vi "Explain Error (Improved) UI.vi"(8 "User VI Ref":refnum<vi>, 9 "Error Cluster":errorcluster) -> ()   [LabVIEW 2020, in "Explain Error Improved Dialog.lvlib"]
uses:
  Explain Error Improved Dialog/Explain Error Improved Dialog.lvlib
  <vilib>/Utility/error.llb/DialogTypeEnum.ctl
  <vilib>/Utility/error.llb/DialogType.ctl
  <vilib>/Platform/browser.llb/Open URL in Default Browser (string).vi
  <vilib>/Utility/inputDevices.llb/mouseAcquire.vi
  <vilib>/Utility/inputDevices.llb/keyboardAcquire.vi
  <vilib>/Utility/cursorutil.llb/Set Cursor (Icon Pict).vi
  <vilib>/Utility/inputDevices.llb/closeKeyboard.vi
  <vilib>/Utility/inputDevices.llb/closeMouse.vi
  fc0d4d85-7f14-4b45-b7f8-c4820347555e.vi
panel:
  in  "search google":bool
  out "Explanation":string
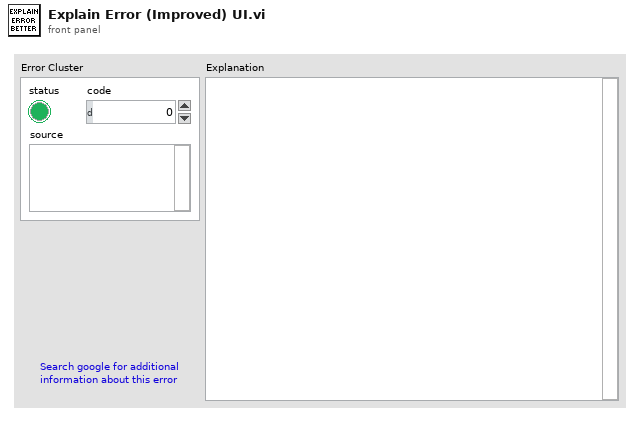
[diagram p1: front panel]
types:
  T1 = typedef "DialogTypeEnum.ctl" = enum16{"no dialog", "OK message", "continue or stop message", "auto error handling dialog", "OK message + warnings", "continue/stop + warnings"}
  T2 = typedef "DialogType.ctl" = u16
  T3 = cluster{"vi name":string, "start":i32, "end":i32}[]
  T4 = typedef "LVPoint32TypeDef.ctl" = cluster{"Horizontal":i32, "Vertical":i32}
  T5 = cluster{"button 1":bool, "button 2":bool, "button 3":bool, "button 4":bool}
  T6 = cluster{"vi name":string, "start":i32, "end":i32}
  T7 = enum16{"0", "1", "2", "3", "4", "5", "6", "7", "8", "9", "A", "B", "C", "D", "E", "F", "G", "H", "I", "J", "K", "L", "M", "N", "O", "P", "Q", "R", "S", "T", "U", "V", "W", "X", "Y", "Z", "F1", "F2", "F3", "F4", "F5", "F6", "F7", "F8", "F9", "F10", "F11", "F12", "F13", "F14", "F15", "ADD", "BACK", "BACKSLASH", "CAPITAL", "COMMA", "DECIMAL", "DELETE", "DIVIDE", "DOWN", "END", "EQUALS", "ESCAPE", "GRAVE (`)", "HOME", "INSERT", "LBRACKET", "LCONTROL", "LEFT", "L ALT", "LSHIFT", "LWIN", "MINUS", "MULTIPLY", "NEXT", "NUMLOCK", "NUMPAD_0", "NUMPAD_1", "NUMPAD_2", "NUMPAD_3", "NUMPAD_4", "NUMPAD_5", "NUMPAD_6", "NUMPAD_7", "NUMPAD_8", "NUMPAD_9", "PAUSE", "PERIOD", "PRIOR (PG UP)", "RBRACKET", "RCONTROL", "RETURN", "RIGHT", "R ALT", "RSHIFT", "RWIN", "SCROLL", "SEMICOLON", "SLASH", "SPACE", "SUBTRACT", "TAB", "UP", "ENTER (num pad)", "' (quote)"}[]
  T8 = cluster{"Shift":bool, "Ctrl":bool, "Alt":bool, "Cmd":bool, "Opt":bool}
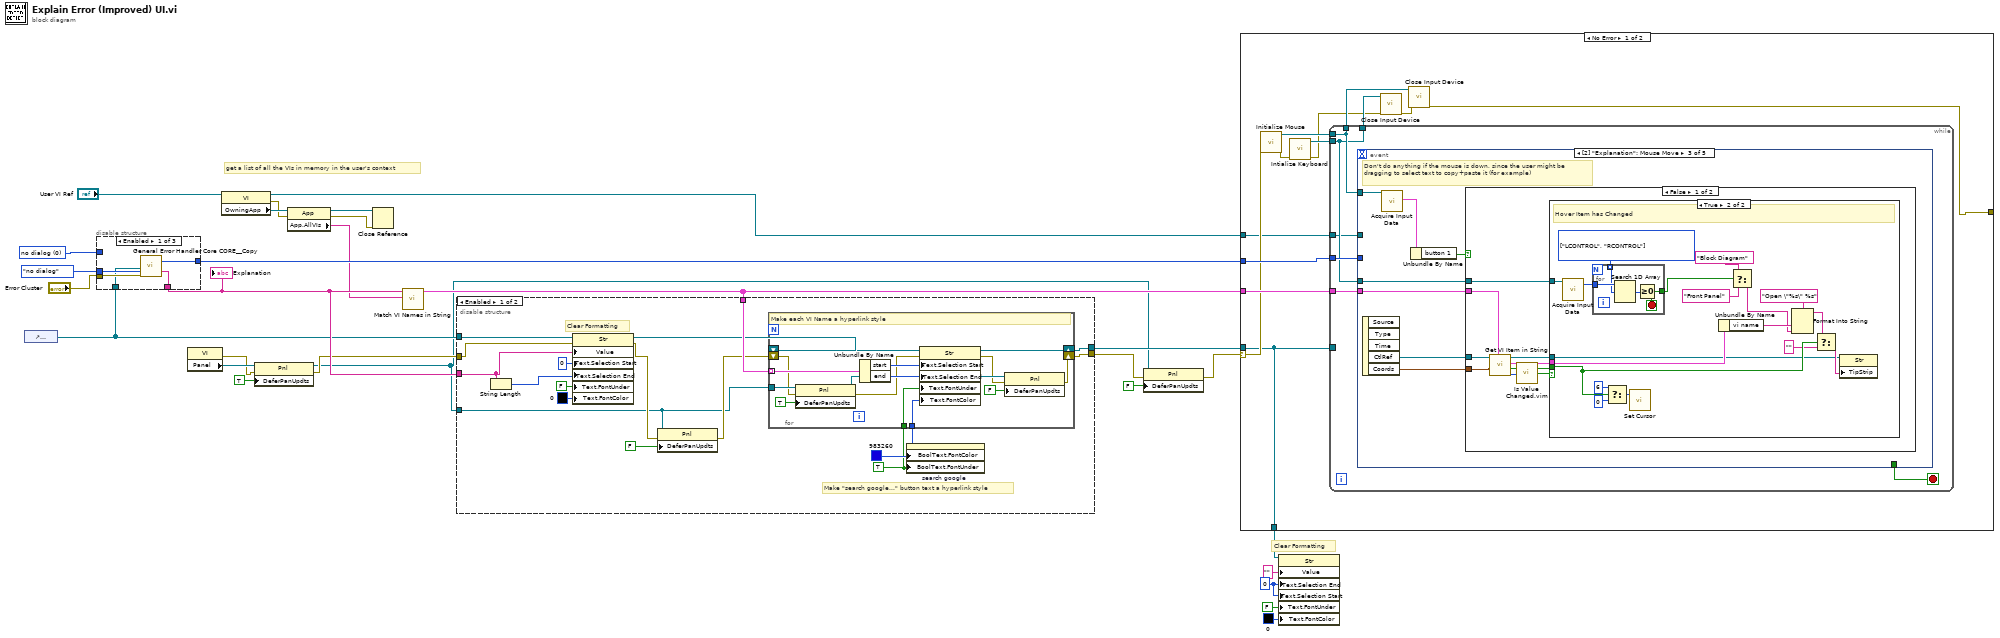
[diagram p0: block diagram]
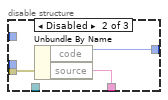
[diagram p3: hidden frame]
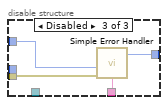
[diagram p4: hidden frame]
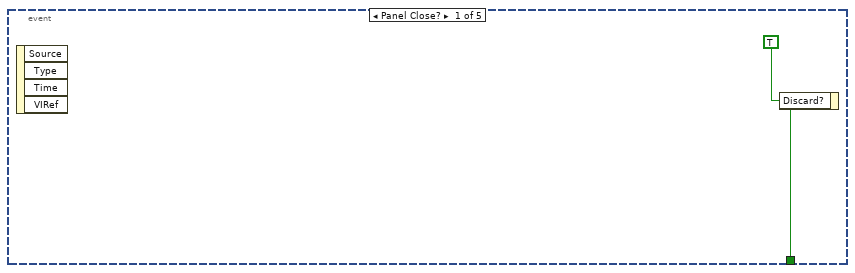
[diagram p5: hidden frame]
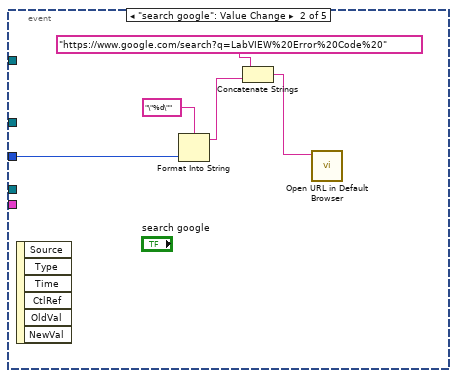
[diagram p6: hidden frame]
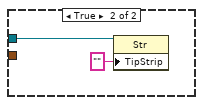
[diagram p8: hidden frame]
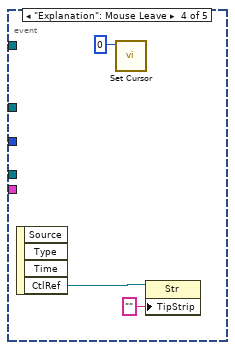
[diagram p9: hidden frame]
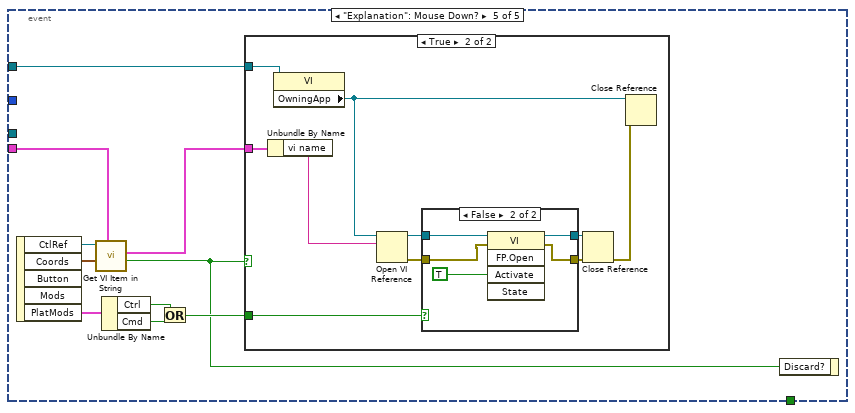
[diagram p10: hidden frame]
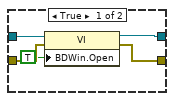
[diagram p12: hidden frame]
diagram:
  w16 = u32 0 ("Text.Selection:End")
  w23 = T2 0 items=["no dialog", "OK message", "continue or stop message", "OK message + warnings", "continue/stop + warnings"] ("type of dialog (OK msg:1)")
  # "get a list of all the VIs in memory in the user's context"
  # "Clear Formatting"
  n1 = control-ref of="Explanation"() -> (w20:refnum<vi>)
  n2 = disable-structure shown="Enabled" {
    disable-tunnel: "Error Cluster" -> [w33 w36 w40]
    disable-tunnel: DialogTypeEnum."no dialog" ("type of dialog (OK msg:1)") -> [w32 _ _]
    disable-tunnel: [w31 w34 w39] -> w21
    disable-tunnel: [w30 w35 w38] -> w25
    disable-tunnel: w23 -> [_ _ w37]
    disable-tunnel: w20 -> [w29 _ _]
    frame Enabled {
      n3 = call "General Error Handler Core CORE__Copy.vi"("String to Format (not a refnum)"=w29, "type of dialog (OK msg:1)"=w32, "error in (no error)"=w33) -> ("code out"=w30:i32, "message"=w31:string)  [unwired: 11 in, 4 out]
    }
    frame Disabled {
      n4 = Unbundle By Name(w36) -> ("code"=w35:i32, "source"=w34:string)
    }
    frame Disabled {
      n5 = call <vilib>:"Simple Error Handler.vi"("type of dialog (OK msg:1)"=w37, "error in (no error)"=w40) -> ("code out"=w38:i32, "message"=w39:string)  [unwired: 3 in, 3 out]
    }
  }
  "Explanation" <- w21
  n6 = property class="VI"() -> (error out=w12:errorcluster, "Panel"=w14:refnum<vi>)  [unwired: 2 in, 1 out]
  n7 = property class="VI"(reference="User VI Ref") -> (reference out=w6:refnum<vi>, error out=w2:errorcluster, "OwningApp"=w5:refnum<vi>)  [unwired: 1 in]
  n8 = property class="Pnl"(reference=w14, error in=w12, "DeferPanUpdts"=TRUE ("Defer Panel Updates")) -> (reference out=w7:refnum<vi>, error out=w8:errorcluster)
  n9 = property class="App"(reference=w5, error in=w2) -> (reference out=w3:refnum<vi>, error out=w1:errorcluster, "App.AllVIs"=w4:string[])
  n10 = Close Reference(reference=w3, error in (no error)=w1) -> ()  [unwired: 1 out]
  n11 = call "Match VI Names in String.vi"("Application:All VIs In Memory"=w4, "string"=w21) -> ("vi names"=w28:T3)  [unwired: 9 in]
  n12 = disable-structure shown="Enabled" {
    disable-tunnel: w28 -> [w57 _]
    disable-tunnel: [w53 w73] -> w27
    disable-tunnel: [w50 _] -> w10
    disable-tunnel: w21 -> [w47 _]
    disable-tunnel: w20 -> [w49 w73]
    disable-tunnel: w8 -> [w48 _]
    disable-tunnel: w7 -> [w41 _]
    frame Enabled {
      w51 = TRUE ("Text.Font:Underline")
      w52 = u32 983260
      # "Make \"search google...\" button text a hyperlink style"
      # "Clear Formatting"
      n13 = String Length(string=w47) -> (length=w46:i32)
      n14 = property class="Str"(reference=w49, error in=w48, "Value"=w47, "Text.Selection Start"=u32 0 ("Text.Selection:Start"), "Text.Selection End"=w46, "Text.FontUnder"=FALSE ("Text.Font:Underline"), "Text.FontColor"=u32 0 ("Text.Font:Color")) -> (reference out=w56:refnum<vi>, error out=w43:errorcluster)
      n15 = property class="Pnl"(reference=w41, error in=w43, "DeferPanUpdts"=FALSE ("Defer Panel Updates")) -> (error out=w42:errorcluster)  [unwired: 1 out]
      n16 = for {
        tunnel: w57 -> [w71] mode=indexing
        shift-right: [w68] -> w53
        shift-left: w56 -> [w72]
        tunnel: w52 -> [w67]
        tunnel: w51 -> [w66]
        shift-right: [w58] -> w50
        shift-left: w42 -> [w60]
        tunnel: w41 -> [w64]
        # "Make each VI Name a hyperlink style"
        n17 = property class="Pnl"(reference=w64, error in=w60, "DeferPanUpdts"=TRUE ("Defer Panel Updates")) -> (reference out=w62:refnum<vi>, error out=w61:errorcluster)
        n18 = Unbundle By Name(w71) -> ("start"=w70:i32, "end"=w69:i32)
        n19 = property class="Str"(reference=w72, error in=w61, "Text.Selection Start"=w70, "Text.Selection End"=w69, "Text.FontUnder"=w66, "Text.FontColor"=w67) -> (reference out=w68:refnum<vi>, error out=w59:errorcluster)
        n20 = property class="Pnl"(reference=w62, error in=w59, "DeferPanUpdts"=FALSE ("Defer Panel Updates")) -> (error out=w58:errorcluster)  [unwired: 1 out]
      }
      n21 = property on="search google" class="Bool (strict)"("BoolText.FontColor"=w52, "BoolText.FontUnder"=w51) -> ()  [unwired: 2 in, 2 out]
    }
    frame Disabled {
    }
  }
  n22 = property class="Pnl"(reference=w7, error in=w10, "DeferPanUpdts"=FALSE ("Defer Panel Updates")) -> (error out=w9:errorcluster)  [unwired: 1 out]
  n23 = case shown="No Error" w9 {
    selector: w9 -> [w80 w173]
    tunnel: w28 -> [w86 _]
    tunnel: w27 -> [w74 w172]
    tunnel: w25 -> [w81 _]
    tunnel: [w75 w173] -> _
    tunnel: w6 -> [w76 _]
    tunnel: [w74 w172] -> w15
    frame No Error {
      n24 = call <vilib>:"Initialize Mouse.vi"("error in (no error)"=w80) -> ("error out"=w79:errorcluster, "device ID"=w85:refnum<k1>)  [unwired: 9 in]
      n25 = call <vilib>:"Intialize Keyboard.vi"("error in (no error)"=w79) -> ("error out"=w78:errorcluster, "device ID"=w83:refnum<k1>)  [unwired: 9 in]
      n26 = while {
        tunnel: w86 -> [w91]
        tunnel: w85 -> [w90]
        tunnel: [w90] -> w84
        tunnel: w74 -> [_]
        tunnel: w81 -> [w89]
        tunnel: w83 -> [w88]
        tunnel: [w88] -> w82
        tunnel: w76 -> [w87]
        stop <- w92 stop-if-true
        n27 = event shown="[2] \"Explanation\": Mouse Move" {
          selector: _ -> [_ _ _ _ _]
          dyn-events: _ -> [_ _ _ _ _]
          timeout: _ -> [_ _ _ _ _]
          tunnel: [w93 _ _ _ _] -> w92
          tunnel: w91 -> [_ _ w104 _ w150]
          tunnel: w90 -> [_ _ w102 _ _]
          tunnel: w89 -> [_ w98 _ _ _]
          tunnel: w88 -> [_ _ w99 _ _]
          tunnel: w87 -> [_ _ _ _ w143]
          event Panel Close? {
            w93 = TRUE ("Discard?")
            n28 = event-data() -> ()  [unwired: 1 in, 4 out]
            n29 = event-data("Discard?"=w93) -> ()  [unwired: 1 in, 1 out]
          }
          event "search google": Value Change {
            n30 = event-data() -> ()  [unwired: 1 in, 6 out]
            n31 = Format Into String(format string="\"%d\"", w98) -> (resulting string=w97:string)  [unwired: 2 in, 1 out]
            n32 = Concatenate Strings("https://www.google.com/search?q=LabVIEW%20Error%20Code%20" ("format string"), w97) -> (w95:string)
            n33 = call-poly <vilib>:"Open URL in Default Browser.vi"("URL"=w95) -> ()  [unwired: 5 in, 2 out]
          }
          event "Explanation": Mouse Move {
            # "Don't do anything if the mouse is down, since the user might be dragging to select text to copy+paste it (for example)"
            n34 = event-data() -> ("CtlRef"=w103:refnum<vi>, "Coords"=w105:T4)  [unwired: 1 in, 3 out]
            n35 = call-poly <vilib>:"Acquire Input Data.vi"("device ID"=w102) -> ("button info"=w101:T5)  [unwired: 15 in, 3 out]
            n36 = Unbundle By Name(w101) -> ("button 1"=w100:bool)
            n37 = case shown="False" w100 {
              tunnel: w105 -> [w114 _]
              tunnel: w104 -> [w113 _]
              tunnel: w103 -> [w110 w138]
              tunnel: w99 -> [w109 _]
              frame False {
                n38 = call "Get VI Item in String.vi"("items"=w113, "Coords"=w114, "String in"=w110) -> ("item index"=w107:i32, "active item"=w111:bool, "item at coords"=w112:T6, "String out"=w108:refnum<vi>)  [unwired: 5 in]
                n39 = call "Is Value Changed.vim"("value"=w107) -> ("changed or first call?"=w106:bool)
                n40 = case shown="True" w106 {
                  tunnel: w112 -> [_ w128]
                  tunnel: w111 -> [_ w117]
                  tunnel: w109 -> [_ w125]
                  tunnel: w108 -> [_ w115]
                  frame False {
                  }
                  frame True {
                    w124 = T7 [enum."LCONTROL", enum."RCONTROL"] items=["0", "1", "2", "3", "4", "5", "6", "7", "8", "9", "A", "B", "C", "D", "E", "F", "G", "H", "I", "J", "K", "L", "M", "N", "O", "P", "Q", "R", "S", "T", "U", "V", "W", "X", "Y", "Z", "F1", "F2", "F3", "F4", "F5", "F6", "F7", "F8", "F9", "F10", "F11", "F12", "F13", "F14", "F15", "ADD", "BACK", "BACKSLASH", "CAPITAL", "COMMA", "DECIMAL", "DELETE", "DIVIDE", "DOWN", "END", "EQUALS", "ESCAPE", "GRAVE (`)", "HOME", "INSERT", "LBRACKET", "LCONTROL", "LEFT", "L ALT", "LSHIFT", "LWIN", "MINUS", "MULTIPLY", "NEXT", "NUMLOCK", "NUMPAD_0", "NUMPAD_1", "NUMPAD_2", "NUMPAD_3", "NUMPAD_4", "NUMPAD_5", "NUMPAD_6", "NUMPAD_7", "NUMPAD_8", "NUMPAD_9", "PAUSE", "PERIOD", "PRIOR (PG UP)", "RBRACKET", "RCONTROL", "RETURN", "RIGHT", "R ALT", "RSHIFT", "RWIN", "SCROLL", "SEMICOLON", "SLASH", "SPACE", "SUBTRACT", "TAB", "UP", "ENTER (num pad)", "' (quote)"] ("keys pressed")
                    # "Hover Item has Changed"
                    n41 = call-poly <vilib>:"Acquire Input Data.vi"("device ID"=w125) -> ("keys pressed"=w123:T7)  [unwired: 16 in, 2 out]
                    n42 = for {
                      tunnel: w124 -> [w135] mode=indexing
                      tunnel: w123 -> [w136]
                      tunnel: [w133] -> w122
                      stop <- w133 stop-if-true
                      n43 = Search 1D Array(1D array=w136, element=w135) -> (index of element=w134:i32)  [unwired: 1 in]
                      n44 = Greater Or Equal To 0?(x=w134) -> (x >= 0?=w133:bool)
                    }
                    n45 = Select(t=u16 6 ("icon"), s=w117, f=u16 0 ("icon")) -> (s? t:f=w130:u16)
                    n46 = call-poly <vilib>:"Set Cursor.vi"("icon"=w130) -> ()  [unwired: 9 in, 2 out]
                    n47 = Unbundle By Name(w128) -> ("vi name"=w127:string)
                    n48 = Select(t="Block Diagram" ("format string"), s=w122, f="Front Panel" ("format string")) -> (s? t:f=w119:string)
                    n49 = Format Into String(format string="Open \"%s\" %s", w127, w119) -> (resulting string=w118:string)  [unwired: 2 in, 1 out]
                    n50 = Select(t=w118, s=w117, f="" ("format string")) -> (s? t:f=w129:string)
                    n51 = property class="Str"(reference=w115, "TipStrip"=w129) -> ()  [unwired: 1 in, 2 out]
                  }
                }
              }
              frame True {
                n52 = property class="Str"(reference=w138, "TipStrip"="" ("Tip Strip")) -> ()  [unwired: 1 in, 2 out]
              }
            }
          }
          event "Explanation": Mouse Leave {
            n53 = event-data() -> ("CtlRef"=w139:refnum<vi>)  [unwired: 1 in, 3 out]
            n54 = call-poly <vilib>:"Set Cursor.vi"("icon"=u16 0) -> ()  [unwired: 9 in, 2 out]
            n55 = property class="Str"(reference=w139, "TipStrip"="" ("Tip Strip")) -> ()  [unwired: 1 in, 2 out]
          }
          event "Explanation": Mouse Down? {
            n56 = event-data() -> ("CtlRef"=w149:refnum<vi>, "Coords"=w151:T4, "PlatMods"=w148:T8)  [unwired: 1 in, 2 out]
            n57 = call "Get VI Item in String.vi"("items"=w150, "Coords"=w151, "String in"=w149) -> ("active item"=w144:bool, "item at coords"=w142:T6)  [unwired: 5 in, 2 out]
            n58 = Unbundle By Name(w148) -> ("Ctrl"=w146:bool, "Cmd"=w147:bool)
            n59 = Or(x=w146, y=w147) -> (x .or. y?=w145:bool)
            n60 = case shown="True" w144 {
              tunnel: w145 -> [_ w157]
              tunnel: w143 -> [_ w154]
              tunnel: w142 -> [_ w156]
              frame False {
              }
              frame True {
                n61 = Unbundle By Name(w156) -> ("vi name"=w155:string)
                n62 = property class="VI"(reference=w154) -> ("OwningApp"=w153:refnum<vi>)  [unwired: 1 in, 2 out]
                n63 = Open VI Reference(application reference (local)=w153, vi path=w155) -> (vi reference=w161:refnum<vi>, error out=w160:errorcluster)  [unwired: 4 in]
                n64 = case shown="False" w157 {
                  tunnel: w161 -> [w166 w171]
                  tunnel: w160 -> [w165 w169]
                  tunnel: [w163 w168] -> w159
                  tunnel: [w162 w167] -> w158
                  frame True {
                    n65 = property class="VI"(reference=w166, error in=w165, "BDWin.Open"=TRUE ("Block Diagram Window:Open")) -> (reference out=w162:refnum<vi>, error out=w163:errorcluster)
                  }
                  frame False {
                    n66 = invoke class="VI" method="FP.Open"(reference=w171, error in=w169, "Activate"=TRUE ("Activate?")) -> (reference out=w167:refnum<vi>, error out=w168:errorcluster)  [unwired: 2 in, 3 out]
                  }
                }
                n67 = Close Reference(reference=w158, error in (no error)=w159) -> (error out=w152:errorcluster)
                n68 = Close Reference(reference=w153, error in (no error)=w152) -> ()  [unwired: 1 out]
              }
            }
            n69 = event-data("Discard?"=w144) -> ()  [unwired: 1 in, 1 out]
          }
        }
      }
      n70 = call-poly <vilib>:"Close Input Device.vi"("error in (no error)"=w78, "device ID"=w82) -> ("error out"=w77:errorcluster)  [unwired: 8 in]
      n71 = call-poly <vilib>:"Close Input Device.vi"("error in (no error)"=w77, "device ID"=w84) -> ("error out"=w75:errorcluster)  [unwired: 8 in]
    }
    frame Error {
    }
  }
  n72 = property class="Str"(reference=w15, "Value"="", "Text.Selection End"=w16, "Text.Selection Start"=w16, "Text.FontUnder"=FALSE ("Text.Font:Underline"), "Text.FontColor"=u32 0 ("Text.Font:Color")) -> ()  [unwired: 1 in, 2 out]
